vi "getConfigArrayByName.vi"(8 "error in (no error)":errorcluster, 10 "device_name":string, 11 "deviceDataBase in":refnum<class "deviceDataBase.lvclass">) -> (0 "error out":errorcluster, 2 "ConfigArray":T1(array[cluster]), 3 "deviceDataBase out":refnum<class "deviceDataBase.lvclass">)   [LabVIEW 2011, in "Tools.lvlib" / "DatabaseHelpers.lvlib" / "deviceDataBase.lvclass"]
uses:
  deviceDataBase.lvclass
  deviceDataBase.lvclass/deviceDataBase.ctl
  Database Objects/device/device.lvclass
  Database Objects/device/EthernetSupply/ethernetSupply.lvclass
  Database Objects/DeviceArray/DeviceArray.lvclass
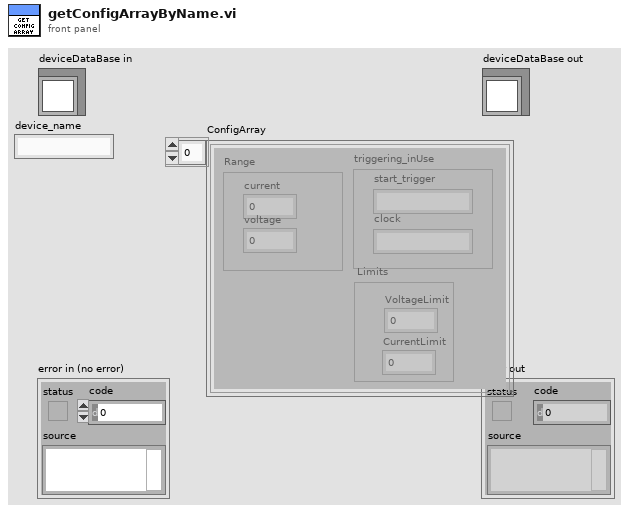
[diagram p1: front panel]
types:
  T1 = cluster{"Range":cluster{"current":dbl, "voltage":dbl}, "triggering_inUse":cluster{"start_trigger":string, "clock":string}, "Limits":cluster{"VoltageLimit":dbl, "CurrentLimit":dbl}}[]
  T2 = cluster{"Range":cluster{"current":dbl, "voltage":dbl}, "triggering_inUse":cluster{"start_trigger":string, "clock":string}, "Limits":cluster{"VoltageLimit":dbl, "CurrentLimit":dbl}}
  T3 = enum16{"digitalOutput", "digitalInput", "analogOutput", "analogInput", "rfOutput", "ethernetSupply"}
  T4 = cluster{"Range":cluster{"units":string, "current":dbl, "voltage":dbl}, "triggering_inUse":cluster{"start_trigger":string, "clock":string}, "Limits":cluster{"VoltageLimit":dbl, "CurrentLimit":dbl}}[]
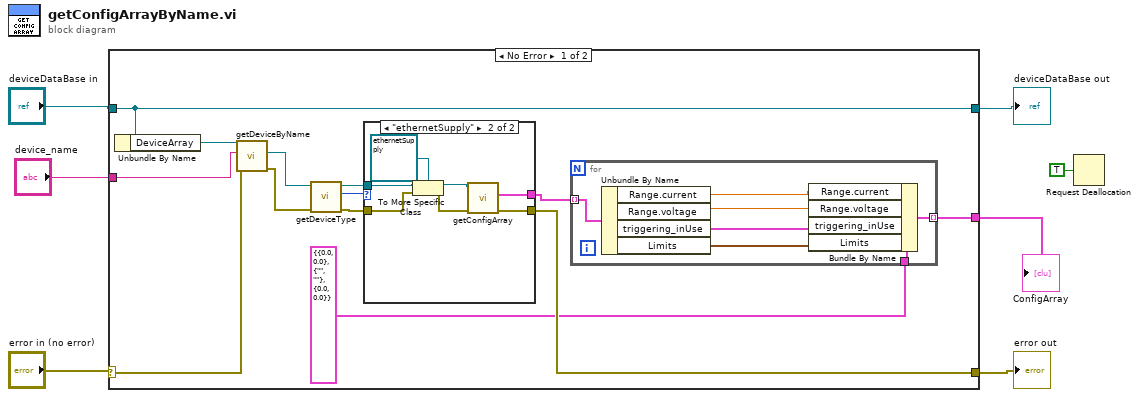
[diagram p0: block diagram]
diagram:
  n1 = case shown="No Error" "error in (no error)" {
    selector: "error in (no error)" -> [w17 w37]
    tunnel: [w11 w37] -> w5
    tunnel: [w20 w36] -> w4
    tunnel: "deviceDataBase in" -> [w20 w36]
    tunnel: "device_name" -> [w18 _]
    tunnel: [w9 _] -> w1
    frame No Error {
      n2 = Unbundle By Name(w20) -> ("DeviceArray"=w19:refnum<class "DeviceArray.lvclass">)
      n3 = call "getDeviceByName.vi"("error in (no error)"=w17, "deviceName"=w18, "DeviceArray in"=w19) -> ("error out"=w15:errorcluster, "device.lvclass"=w16:refnum<class "device.lvclass">)  [unwired: 5 in, 2 out]
      n4 = call-dynamic "getDeviceType.vi"("error in (no error)"=w15, "device.lvclass in"=w16) -> ("error out"=w12:errorcluster, "type"=w14:T3, "device.lvclass out"=w13:refnum<class "device.lvclass">)  [unwired: 7 in]
      n5 = case shown="\"ethernetSupply\"" w14 {
        tunnel: w13 -> [_ w35]
        tunnel: w12 -> [w28 w34]
        tunnel: [w28 w32] -> w11
        tunnel: [_ w29] -> w10
        frame Default {
        }
        frame "ethernetSupply" {
          n6 = To More Specific Class(target class=refnum<class "ethernetSupply.lvclass"> refnum ("Tools.lvlib:DatabaseHelpers.lvlib:EthernetSupply.lvclass"), reference=w35, error in=w34) -> (specific class reference=w30:refnum<class "ethernetSupply.lvclass">, error out=w31:errorcluster)
          n7 = call "getConfigArray.vi"("error in (no error)"=w31, "EthernetSupply in"=w30) -> ("error out"=w32:errorcluster, "ConfigArray"=w29:T4)  [unwired: 7 in, 1 out]
        }
      }
      n8 = for {
        tunnel: w10 -> [w27] mode=indexing
        tunnel: T2 {"Range"={"current"=0.0, "voltage"=0.0}, "triggering_inUse"={"start_trigger"="", "clock"=""}, "Limits"={"VoltageLimit"=0.0, "CurrentLimit"=0.0}} ("channelConfig") -> [w21]
        tunnel: [w22] -> w9 mode=indexing
        n9 = Unbundle By Name(w27) -> ("Range.current"=w24:dbl, "Range.voltage"=w23:dbl, "triggering_inUse"=w25:cluster{"start_trigger":string, "clock":string}, "Limits"=w26:cluster{"VoltageLimit":dbl, "CurrentLimit":dbl})
        n10 = Bundle By Name(cluster=w21, "Range.current"=w24, "Range.voltage"=w23, "triggering_inUse"=w25, "Limits"=w26) -> (w22:T2)
      }
    }
    frame Error {
    }
  }
  "error out" <- w5
  "deviceDataBase out" <- w4
  "ConfigArray" <- w1
  n11 = Request Deallocation(TRUE ("flag")) -> ()
